vi "CH1_Comm.vi"() -> ()   [LabVIEW 2018]
uses:
  Stream/Stream.lvclass
  RxTx/RxTx.lvclass
  Stream/Stream.lvclass/Stream.ctl
panel:
  in  "IP: 2":string="localhost"
  in  "Channel:":u16=1
  in  "IP:":string="localhost"
  in  "RxTx.lvclass 2":refnum<class "RxTx.lvclass">
  in  "Stream.lvclass 2":refnum<class "Stream.lvclass">
  in  "RxTx.lvclass":refnum<class "RxTx.lvclass">
  in  "Stream.lvclass":refnum<class "Stream.lvclass">
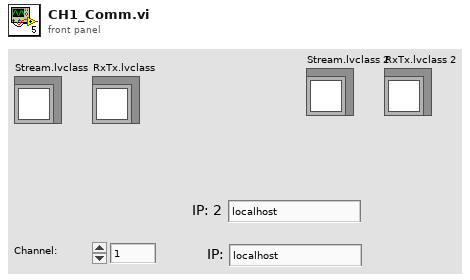
[diagram p1: front panel]
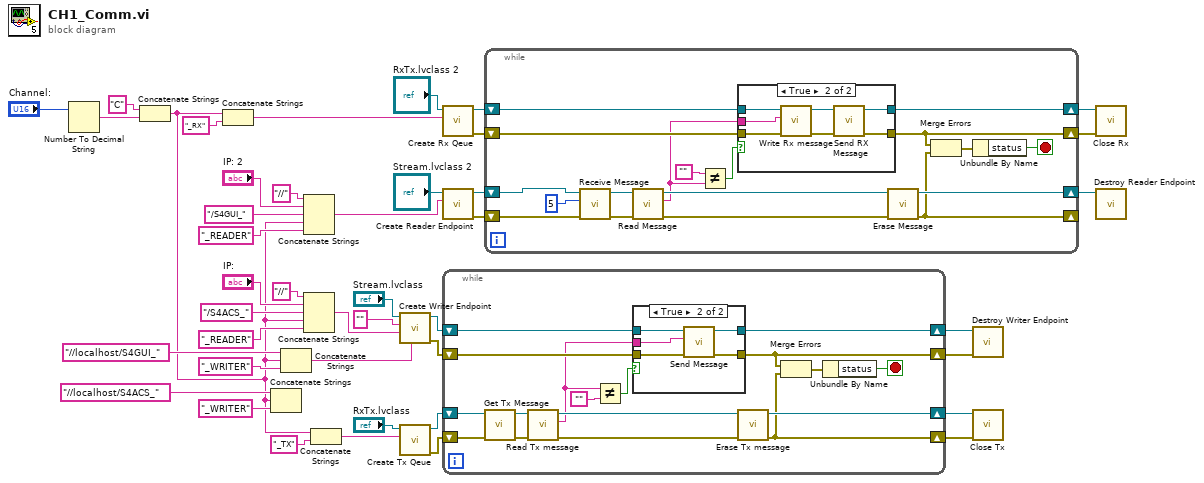
[diagram p0: block diagram]
diagram:
  n1 = Number To Decimal String(number="Channel:") -> (decimal integer string=w13:string)  [unwired: 1 in]
  n2 = Concatenate Strings("C", w13) -> (w6:string)
  n3 = Concatenate Strings(w6, "_RX" ("Reader Name")) -> (w5:string)
  n4 = Concatenate Strings("//localhost/S4ACS_" ("reader name"), w6, "_WRITER" ("reader name")) -> ()  [unwired: 1 out]
  n5 = Concatenate Strings("//localhost/S4GUI_" ("reader name"), w6, "_WRITER" ("reader name")) -> (w1:string)
  n6 = Concatenate Strings("//" ("Reader Name"), "IP: 2", "/S4GUI_" ("Reader Name"), w6, "_READER" ("Reader Name")) -> (w3:string)
  n7 = Concatenate Strings("//" ("Reader Name"), "IP:", "/S4ACS_" ("Reader Name"), w6, "_READER" ("Reader Name")) -> (w2:string)
  n8 = Concatenate Strings(w6, "_TX" ("Reader Name")) -> (w4:string)
  n9 = call "Create Writer Endpoint.vi"("writer name"=w1, "reader name"=w2, "IP"="" ("Reader Name"), "Stream in"="Stream.lvclass") -> ("error out"=w35:errorcluster, "Stream out"=w37:refnum<class "Stream.lvclass">)  [unwired: 6 in]
  n10 = call "Create Tx Qeue.vi"("Writer Name"=w4, "RxTx in"="RxTx.lvclass") -> ("error out"=w41:errorcluster, "RxTx out"=w42:refnum<class "RxTx.lvclass">)  [unwired: 8 in]
  n11 = call "Create Rx Qeue.vi"("Reader Name"=w5, "RxTx in"="RxTx.lvclass 2") -> ("error out"=w26:errorcluster, "RxTx out"=w27:refnum<class "RxTx.lvclass">)  [unwired: 8 in]
  n12 = call "Create Reader Endpoint.vi"("reader name"=w3, "Stream in"="Stream.lvclass 2") -> ("error out"=w30:errorcluster, "Stream out"=w31:refnum<class "Stream.lvclass">)  [unwired: 8 in]
  n13 = while {
    shift-right: [w52] -> w34
    shift-left: w35 -> [w54]
    shift-right: [w53] -> w43
    shift-left: w37 -> [w55]
    shift-right: [w47] -> w38
    shift-left: w41 -> [w56]
    shift-right: [w49] -> w39
    shift-left: w42 -> [w57]
    stop <- w46 stop-if-true
    n14 = call "Get Tx Message.vi"("error in (no error)"=w56, "RxTx in"=w57) -> ("error out"=w59:errorcluster, "RxTx out"=w58:refnum<class "RxTx.lvclass">)  [unwired: 8 in]
    n15 = call "Read Tx message.vi"("error in (no error)"=w59, "RxTx in"=w58) -> ("error out"=w48:errorcluster, "Tx Message"=w45:string, "RxTx out"=w50:refnum<class "RxTx.lvclass">)  [unwired: 7 in]
    n16 = Not Equal?(x=w45, y="") -> (x != y?=w44:bool)
    n17 = case shown="True" w44 {
      tunnel: w55 -> [w62 w67]
      tunnel: w54 -> [w61 w66]
      tunnel: [w62 w65] -> w53
      tunnel: w45 -> [_ w64]
      tunnel: [w61 w63] -> w52
      frame False {
      }
      frame True {
        n18 = call "Send Message.vi"("error in (no error)"=w66, "Message"=w64, "Stream in"=w67) -> ("error out"=w63:errorcluster, "Stream out"=w65:refnum<class "Stream.lvclass">)  [unwired: 7 in]
      }
    }
    n19 = call "Erase Tx message.vi"("error in (no error)"=w48, "RxTx in"=w50) -> ("error out"=w47:errorcluster, "RxTx out"=w49:refnum<class "RxTx.lvclass">)  [unwired: 8 in]
    n20 = Merge Errors(w52, w47) -> (w60:errorcluster)
    n21 = Unbundle By Name(w60) -> ("status"=w46:bool)
  }
  n22 = while {
    shift-right: [w71] -> _
    shift-left: w30 -> [w84]
    shift-right: [w74] -> w29
    shift-left: w31 -> [w85]
    shift-right: [w78] -> w24
    shift-left: w26 -> [w81]
    shift-right: [w80] -> w25
    shift-left: w27 -> [w69]
    stop <- w70 stop-if-true
    n23 = call "Receive Message.vi"("error in (no error)"=w84, "timeout ms"=5, "Stream in"=w85) -> ("error out"=w82:errorcluster, "Stream out"=w83:refnum<class "Stream.lvclass">)  [unwired: 7 in]
    n24 = call "Read Message.vi"("error in (no error)"=w82, "Stream in"=w83) -> ("error out"=w73:errorcluster, "Message"=w68:string, "Stream out"=w72:refnum<class "Stream.lvclass">)  [unwired: 7 in]
    n25 = Not Equal?(x="", y=w68) -> (x != y?=w75:bool)
    n26 = case shown="True" w75 {
      tunnel: w81 -> [w86 w92]
      tunnel: w69 -> [w87 w91]
      tunnel: w68 -> [_ w90]
      tunnel: [w87 w89] -> w80
      tunnel: [w86 w88] -> w78
      frame False {
      }
      frame True {
        n27 = call "Write Rx message.vi"("error in (no error)"=w92, "Rx message"=w90, "RxTx in"=w91) -> ("error out"=w93:errorcluster, "RxTx out"=w94:refnum<class "RxTx.lvclass">)  [unwired: 7 in]
        n28 = call "Send RX Message.vi"("error in (no error)"=w93, "RxTx in"=w94) -> ("error out"=w88:errorcluster, "RxTx out"=w89:refnum<class "RxTx.lvclass">)  [unwired: 8 in]
      }
    }
    n29 = call "Erase Message.vi"("error in (no error)"=w73, "Stream in"=w72) -> ("error out"=w71:errorcluster, "Stream out"=w74:refnum<class "Stream.lvclass">)  [unwired: 8 in]
    n30 = Merge Errors(w78, w71) -> (w79:errorcluster)
    n31 = Unbundle By Name(w79) -> ("status"=w70:bool)
  }
  n32 = call "Destroy Writer Endpoint.vi"("error in (no error)"=w34, "Stream in"=w43) -> ()  [unwired: 8 in, 2 out]
  n33 = call "Close Tx.vi"("error in (no error)"=w38, "RxTx in"=w39) -> ()  [unwired: 8 in, 2 out]
  n34 = call "Close Rx.vi"("error in (no error)"=w24, "RxTx in"=w25) -> ()  [unwired: 8 in, 2 out]
  n35 = call "Destroy Reader Endpoint.vi"("Stream in"=w29) -> ()  [unwired: 9 in, 2 out]
